vi "Boxplot - Compute Whiskers.vi"(9 "Median":dbl format="%#.6g", 10 "Lower quartile (LQ)":dbl format="%#.6g", 11 "Upper quartile (UQ)":dbl format="%#.6g") -> (0 "L2":dbl format="%#.6g", 1 "L1":dbl format="%#.6g", 2 "U1":dbl format="%#.6g", 3 "U2":dbl format="%#.6g")   [LabVIEW 2023]
doc: "Computes the length of the whiskers of the boxplot."
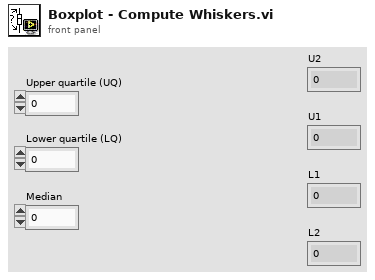
[diagram p1: front panel]
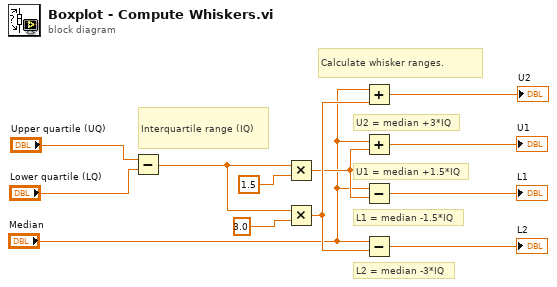
[diagram p0: block diagram]
diagram:
  # "L1 = median -1.5*IQ"
  # "Interquartile range (IQ)"
  # "L2 = median -3*IQ"
  # "U1 = median +1.5*IQ"
  # "U2 = median +3*IQ"
  # "Calculate whisker ranges."
  n1 = Subtract(x="Upper quartile (UQ)", y="Lower quartile (LQ)") -> (x-y=w7:dbl)
  n2 = Multiply(x=w7, y=1.5) -> (x*y=w6:dbl)
  n3 = Multiply(x=w7, y=3.0) -> (x*y=w8:dbl)
  n4 = Add(x="Median", y=w8) -> (x+y=→"U2":dbl)
  n5 = Add(x="Median", y=w6) -> (x+y=→"U1":dbl)
  n6 = Subtract(x="Median", y=w6) -> (x-y=→"L1":dbl)
  n7 = Subtract(x="Median", y=w8) -> (x-y=→"L2":dbl)
